vi "Signal_Hound_Scalar_Network_Analyzer.vi"   [LabVIEW 2024]
uses:
  <instrlib>/Signal Hound SA Series/Signal Hound SA Series.lvlib
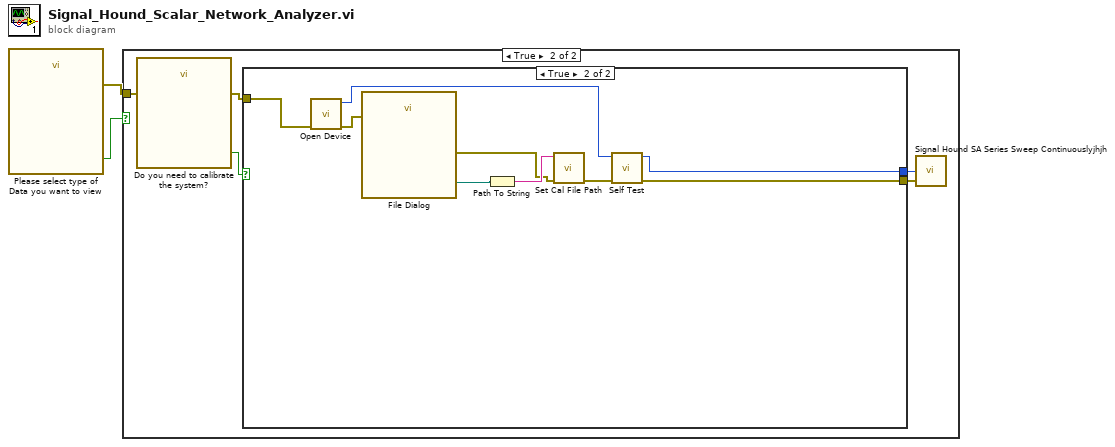
[diagram p0: block diagram]
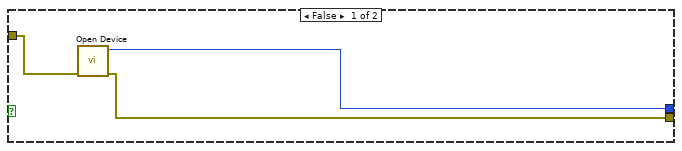
[diagram p3: hidden frame]
diagram:
  n1 = call "Please select type of Data you want to view"() -> ("Live Data"=w2:bool, "error out"=w1:errorcluster)  [unwired: 18 in]
  n2 = case shown="True" w2 {
    tunnel: w1 -> [_ w7]
    frame False {
    }
    frame True {
      n3 = call "Do you need to calibrate the system?"("error in (no error)"=w7) -> ("Yes"=w6:bool, "error out"=w5:errorcluster)  [unwired: 17 in]
      n4 = case shown="True" w6 {
        tunnel: w5 -> [w10 w18]
        tunnel: [w8 w12] -> w4
        tunnel: [w9 w11] -> w3
        frame False {
          n5 = call <instrlib>:"Open Device.vi"("error in (no error)"=w10) -> ("error out"=w8:errorcluster, "device"=w9:i32)  [unwired: 9 in]
        }
        frame True {
          n6 = call <instrlib>:"Open Device.vi"("error in (no error)"=w18) -> ("error out"=w14:errorcluster, "device"=w13:i32)  [unwired: 9 in]
          n7 = call "File Dialog"("error in"=w14) -> ("selected path"=w17:path, "error out"=w15:errorcluster)  [unwired: 11 in, 2 out]
          n8 = Path To String(path=w17) -> (string=w16:string)
          n9 = call <instrlib>:"Set Cal File Path.vi"("error in (no error)"=w15, "path"=w16) -> ("error out"=w19:errorcluster)  [unwired: 9 in]
          n10 = call <instrlib>:"Self Test.vi"("error in (no error)"=w19, "device"=w13) -> ("error out"=w12:errorcluster, "device out"=w11:i32)  [unwired: 7 in, 1 out]
        }
      }
      n11 = call "Signal Hound SA Series Sweep Continuouslyjhjh.vi"("error in (no error)"=w4, "device"=w3) -> ()  [unwired: 1 in]
    }
  }
